vi "RM.getReservationList.vi"(7 "Resource Type":T1, 8 "error in":errorcluster, 11 "reservation DB in":variant) -> (0 "error out":errorcluster, 1 "clientGUIDs":string[](array[string]), 2 "names in bitfile":string[](array[string]), 3 "reservation DB out":variant)   [LabVIEW 2016, in "FPGA Resource Manager.lvlib"]
uses:
  FPGA Resource Manager.lvlib
  RM.resourceType.ctl
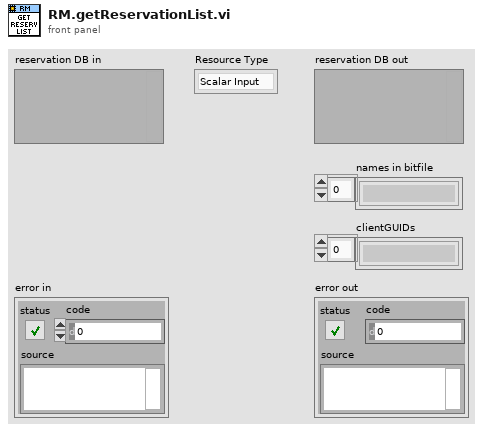
[diagram p1: front panel]
types:
  T1 = typedef "FPGA Resource Manager.lvlib/RM.resourceType.ctl" = enum16{"Scalar Input", "Scalar Output", "Waveform Input", "Waveform Output"}
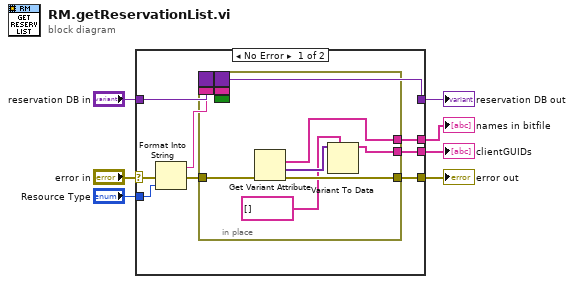
[diagram p0: block diagram]
diagram:
  n1 = case shown="No Error" "error in" {
    selector: "error in" -> [w11 w25]
    tunnel: "reservation DB in" -> [w16 w26]
    tunnel: [w15 w26] -> w3
    tunnel: "Resource Type" -> [w14 _]
    tunnel: [w10 w25] -> w4
    tunnel: [w9 _] -> w2
    tunnel: [w8 _] -> w1
    frame No Error {
      n2 = Format Into String(error in=w11, w14) -> (resulting string=w13:string, error out=w12:errorcluster)  [unwired: 2 in]
      n3 = in-place {
        in-place-border: w12 -> [w24]
        in-place-border: [w23] -> w10
        in-place-border: [w22] -> w9
        border: w16 -> [_]
        border: w13 -> [_]
        border: [_] -> w15
        border: _ -> [_]
        border: _ -> [_]
        in-place-border: [w21] -> w8
        n4 = Get Variant Attribute(Variant=w18, error in=w24) -> (duplicate Variant=w17:variant, names=w22:string[], values=w20:variant[], error out=w23:errorcluster)  [unwired: 2 in]
        n5 = Variant To Data(type=string[] [] ("name"), Variant=w20) -> (data=w21:string[])  [unwired: 1 in, 1 out]
      }
    }
    frame Error {
    }
  }
  "reservation DB out" <- w3
  "error out" <- w4
  "names in bitfile" <- w2
  "clientGUIDs" <- w1
